vi "RSZVB Get Sweep Segment Bit Values.vi"(8 "error in (no error)":errorcluster {"code" format="%.0x"}, 9 "Segment (1)":i32=1, 10 "Channel (1)":i32=1, 11 "VISA session":refnum<visa-resource-name>) -> (0 "error out":errorcluster {"code" format="%.0x"}, 1 "Bit 3":bool, 2 "Bit 2":bool, 3 "dup VISA session":refnum<visa-resource-name>, 5 "Bit 1":bool, 7 "Bit 0":bool)   [LabVIEW 2011]
doc: "This VI returns four independent output signals at the USER CONTROL connector (lines 8, 9, 10, 11). \n\nOUTPut<Ch>:UPORt:SEGMent<Seg>[:VALue]?"
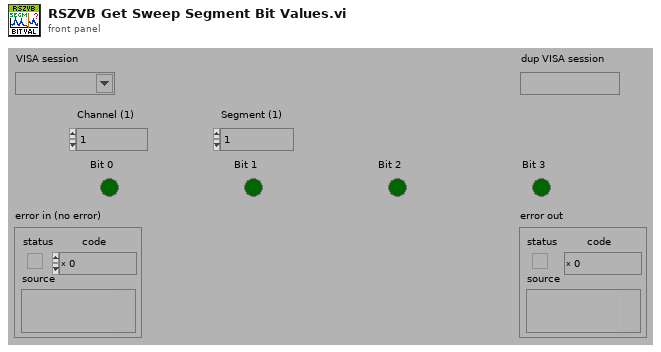
[diagram p1: front panel]
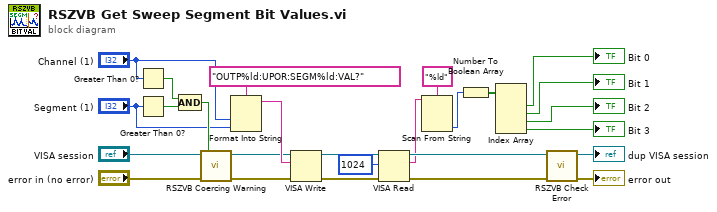
[diagram p0: block diagram]
diagram:
  n1 = Greater Than 0?(x="Channel (1)") -> (x > 0?=w24:bool)
  n2 = Greater Than 0?(x="Segment (1)") -> (x > 0?=w25:bool)
  n3 = Compound Arithmetic op=AND(w24, w25) -> (w23:bool)
  n4 = call "RSZVB Coercing Warning.vi"("In Range?"=w23, "error in (no error)"="error in (no error)", "VISA session"="VISA session") -> ("error out"=w22:errorcluster, "dup VISA session"=w21:refnum<visa-resource-name>)  [unwired: 7 in]
  n5 = Format Into String(format string="OUTP%ld:UPOR:SEGM%ld:VAL?", "Channel (1)", "Segment (1)") -> (resulting string=w26:string)  [unwired: 2 in, 1 out]
  n6 = VISA Write(VISA resource name=w21, write buffer=w26, error in (no error)=w22) -> (VISA resource name out=w11:refnum<visa-resource-name>, error out=w12:errorcluster)  [unwired: 1 out]
  n7 = VISA Read(VISA resource name=w11, byte count=u32 1024 ("byte count (0)"), error in (no error)=w12) -> (VISA resource name out=w7:refnum<visa-resource-name>, read buffer=w5:string, error out=w6:errorcluster)  [unwired: 1 out]
  n8 = Scan From String(format string="%ld", input string=w5) -> (output 1=w9:i32)  [unwired: 3 in, 3 out]
  n9 = Number To Boolean Array(number=w9) -> (Boolean array=w8:bool[])
  n10 = Index Array(array=w8) -> (element #1=→"Bit 0":bool, element #2=→"Bit 1":bool, element #3=→"Bit 2":bool, element #4=→"Bit 3":bool)  [unwired: 4 in]
  n11 = call "RSZVB Check Error.vi"("error in (no error)"=w6, "VISA session"=w7) -> ("error out"=→"error out":errorcluster, "dup VISA session"=→"dup VISA session":refnum<visa-resource-name>)  [unwired: 8 in]
